vi "License Generator.vi"() -> ()   [LabVIEW 2019]
panel:
  in  "SP Generate":bool
  out "SP":string caption="Swelling Pressure"
  in  "Client MAC Address":string caption="Triaxial Shear 2"
  in  "Iso Generate":bool
  in  "UCT Generate":bool
  in  "Sat Generate":bool
  in  "Cons Generate":bool
  in  "Permeability Generate":bool
  in  "Shearbox Generate":bool
  in  "TUU Generate":bool
  in  "TS Generate":bool
  out "Isotropic":string caption="Isotropic Consolidation"
  out "UCT":string
  out "Saturation":string caption="Saturation (Incremental)"
  out "Consolidation":string caption="Consolidation (Stepped Loadning)"
  out "Permeability":string
  out "Shearbox":string
  out "Triaxial UU":string
  out "Triaxial Shear":string
  # "\"getmac\" on client command prompt"
  # "Test Type Module"
  # "Activation Code"
  # "Generate"
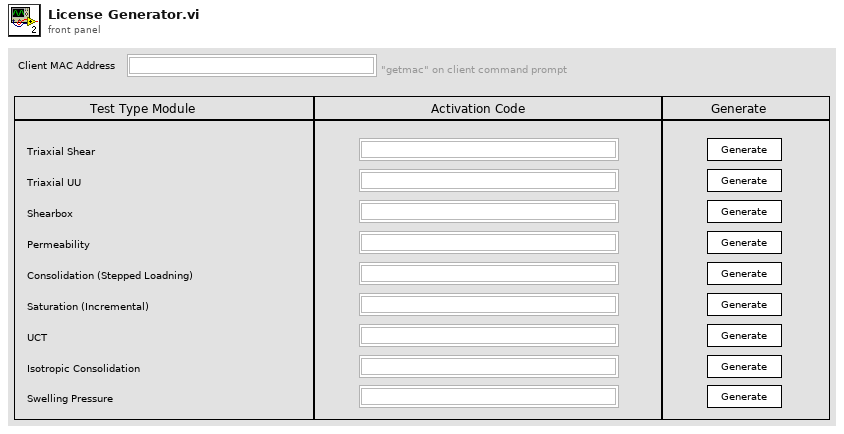
[diagram p1: front panel]
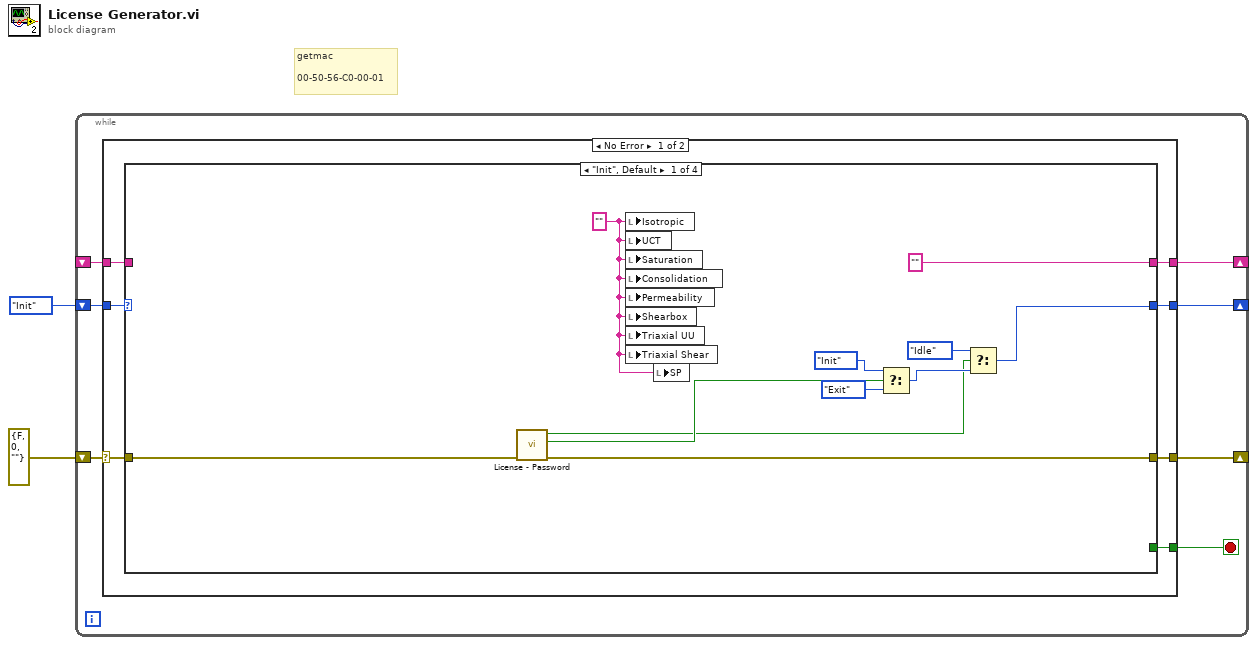
[diagram p0: block diagram]
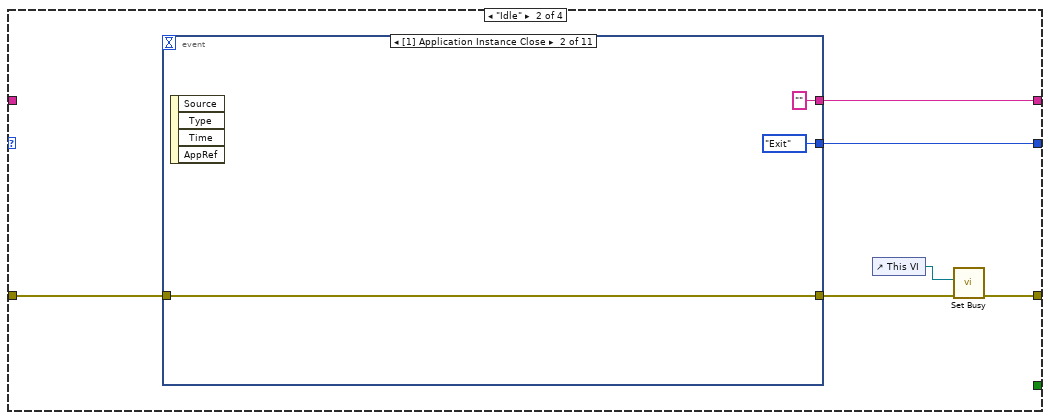
[diagram p2: hidden frame]
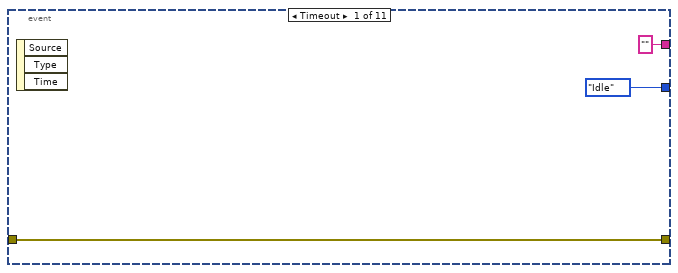
[diagram p3: hidden frame]
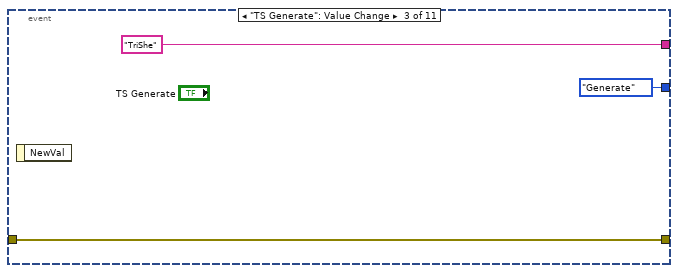
[diagram p4: hidden frame]
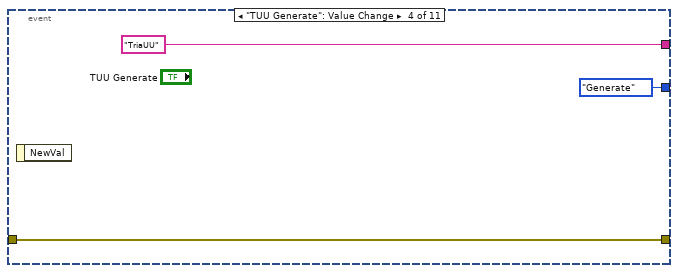
[diagram p5: hidden frame]
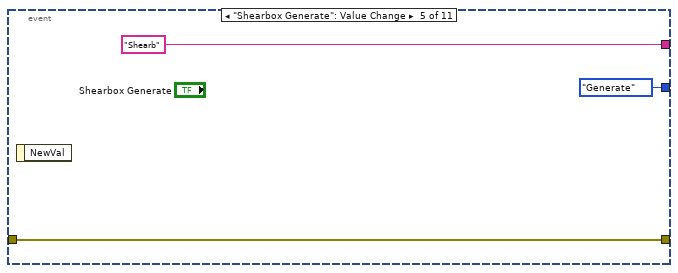
[diagram p6: hidden frame]
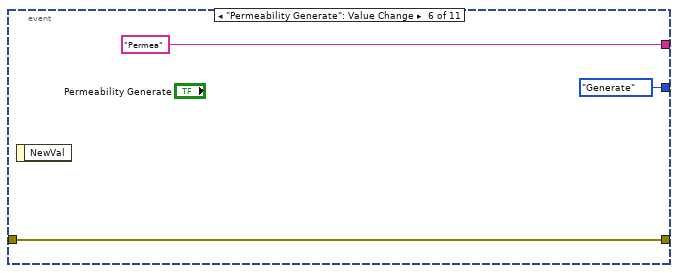
[diagram p7: hidden frame]
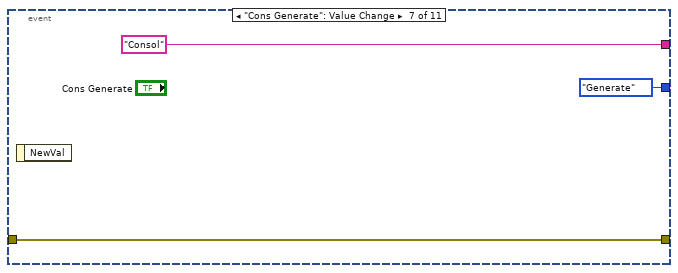
[diagram p8: hidden frame]
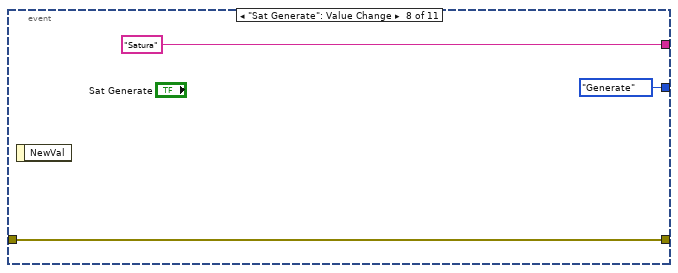
[diagram p9: hidden frame]
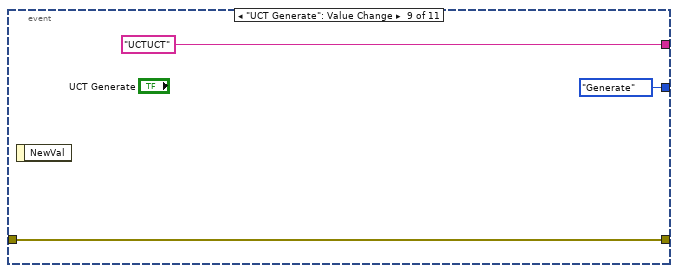
[diagram p10: hidden frame]
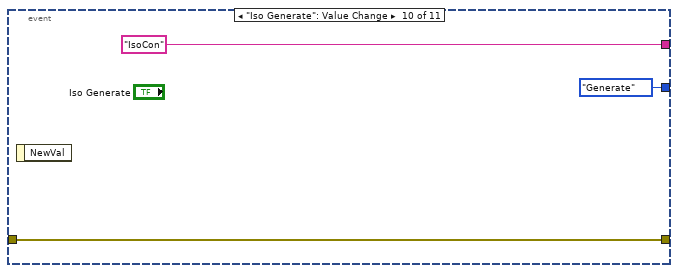
[diagram p11: hidden frame]
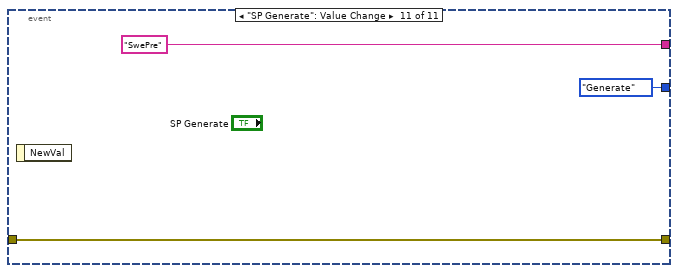
[diagram p12: hidden frame]
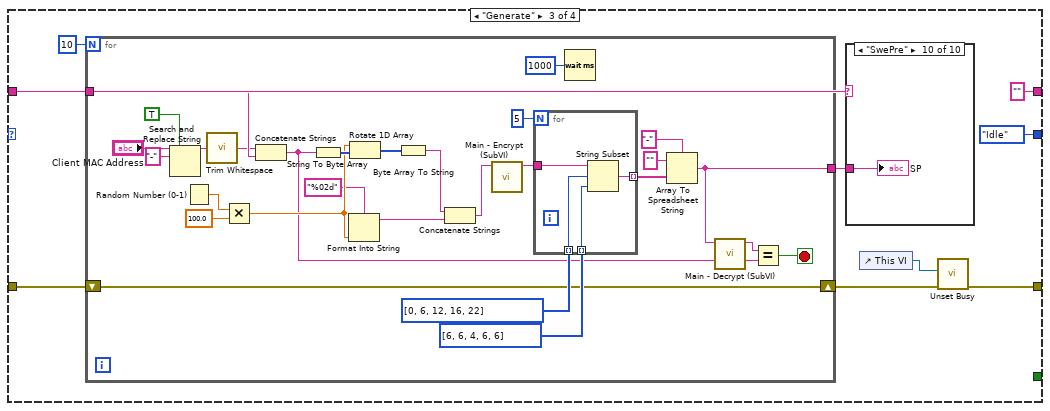
[diagram p13: hidden frame]
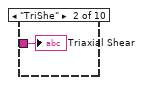
[diagram p15: hidden frame]
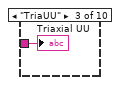
[diagram p16: hidden frame]
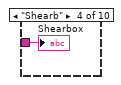
[diagram p17: hidden frame]
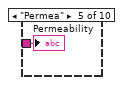
[diagram p18: hidden frame]
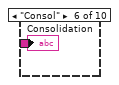
[diagram p19: hidden frame]
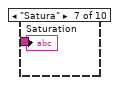
[diagram p20: hidden frame]
diagram:
  # "getmac\n\n00-50-56-C0-00-01"
  n1 = while {
    shift-right: [w6] -> _
    shift-left: enum16{"Init", "Idle", "Generate", "Exit"}."Init" -> [w9]
    shift-right: [w7] -> _
    shift-left: errorcluster {"status"=FALSE, "code"=0, "source"=""} ("error constant") -> [w8]
    shift-right: [w5] -> _
    shift-left: _ -> [w4]
    stop <- w3 stop-if-true
    n2 = case shown="No Error" w8 {
      selector: w8 -> [w14 w125]
      tunnel: w9 -> [w16 _]
      tunnel: [w15 w124] -> w7
      tunnel: [w13 enum16{"Init", "Idle", "Generate", "Exit"}."Idle"] -> w6
      tunnel: [w12 ""] -> w5
      tunnel: w4 -> [w11 _]
      tunnel: [w10 _] -> w3
      frame No Error {
        n3 = case shown="\"Init\", Default" w16 {
          tunnel: [w25 w30 w68 w120] -> w15
          tunnel: w14 -> [w24 w33 w70 w120]
          tunnel: [w17 w32 enum16{"Init", "Idle", "Generate", "Exit"}."Idle" enum16{"Init", "Idle", "Generate", "Exit"}."Exit"] -> w13
          tunnel: ["" w31 "" ""] -> w12
          tunnel: w11 -> [_ _ w73 _]
          tunnel: [_ _ _ TRUE] -> w10
          frame "Init", Default {
            w26 = "" ("Isotropic")
            n4 = call "License - Password.vi"("error in"=w24) -> ("error out"=w25:errorcluster, "T button?"=w23:bool, "Pass?"=w19:bool)  [unwired: 8 in]
            n5 = local write "Isotropic"(w26) -> ()
            n6 = local write "UCT"(w26) -> ()
            n7 = local write "Saturation"(w26) -> ()
            n8 = local write "Consolidation"(w26) -> ()
            n9 = local write "Permeability"(w26) -> ()
            n10 = local write "Shearbox"(w26) -> ()
            n11 = local write "Triaxial UU"(w26) -> ()
            n12 = local write "Triaxial Shear"(w26) -> ()
            n13 = local write "SP"(w26) -> ()
            n14 = Select(t=enum16{"Init", "Idle", "Generate", "Exit"}."Init", s=w23, f=enum16{"Init", "Idle", "Generate", "Exit"}."Exit") -> (s? t:f=w20:enum16{"Init", "Idle", "Generate", "Exit"})
            n15 = Select(t=enum16{"Init", "Idle", "Generate", "Exit"}."Idle", s=w19, f=w20) -> (s? t:f=w17:enum16{"Init", "Idle", "Generate", "Exit"})
          }
          frame "Idle" {
            n16 = event shown="[1] Application Instance Close" {
              selector: _ -> [_ _ _ _ _ _ _ _ _ _ _]
              dyn-events: _ -> [_ _ _ _ _ _ _ _ _ _ _]
              timeout: _ -> [_ _ _ _ _ _ _ _ _ _ _]
              tunnel: [w36 w39 w42 w45 w48 w51 w54 w57 w60 w63 w66] -> w29
              tunnel: w33 -> [w36 w39 w42 w45 w48 w51 w54 w57 w60 w63 w66]
              tunnel: [enum16{"Init", "Idle", "Generate", "Exit"}."Idle" enum16{"Init", "Idle", "Generate", "Exit"}."Exit" enum16{"Init", "Idle", "Generate", "Exit"}."Generate" enum16{"Init", "Idle", "Generate", "Exit"}."Generate" enum16{"Init", "Idle", "Generate", "Exit"}."Generate" enum16{"Init", "Idle", "Generate", "Exit"}."Generate" enum16{"Init", "Idle", "Generate", "Exit"}."Generate" enum16{"Init", "Idle", "Generate", "Exit"}."Generate" enum16{"Init", "Idle", "Generate", "Exit"}."Generate" enum16{"Init", "Idle", "Generate", "Exit"}."Generate" enum16{"Init", "Idle", "Generate", "Exit"}."Generate"] -> w32
              tunnel: ["" "" "TriShe" "TriaUU" "Shearb" "Permea" "Consol" "Satura" "UCTUCT" "IsoCon" "SwePre"] -> w31
              event Timeout {
                n17 = event-data() -> ()  [unwired: 1 in, 3 out]
              }
              event Application Instance Close {
                n18 = event-data() -> ()  [unwired: 1 in, 4 out]
              }
              event "TS Generate": Value Change {
                n19 = event-data() -> ()  [unwired: 1 in, 1 out]
              }
              event "TUU Generate": Value Change {
                n20 = event-data() -> ()  [unwired: 1 in, 1 out]
              }
              event "Shearbox Generate": Value Change {
                n21 = event-data() -> ()  [unwired: 1 in, 1 out]
              }
              event "Permeability Generate": Value Change {
                n22 = event-data() -> ()  [unwired: 1 in, 1 out]
              }
              event "Cons Generate": Value Change {
                n23 = event-data() -> ()  [unwired: 1 in, 1 out]
              }
              event "Sat Generate": Value Change {
                n24 = event-data() -> ()  [unwired: 1 in, 1 out]
              }
              event "UCT Generate": Value Change {
                n25 = event-data() -> ()  [unwired: 1 in, 1 out]
              }
              event "Iso Generate": Value Change {
                n26 = event-data() -> ()  [unwired: 1 in, 1 out]
              }
              event "SP Generate": Value Change {
                n27 = event-data() -> ()  [unwired: 1 in, 1 out]
              }
            }
            n28 = control-ref of="This VI"() -> (w28:refnum<vi>)
            n29 = call <vilib>:"Set Busy.vi"("error in (no error)"=w29, "VI reference (current VI)"=w28) -> ("error out"=w30:errorcluster)  [unwired: 8 in, 1 out]
          }
          frame "Generate" {
            n30 = for {
              N: 10 -> [_]
              tunnel: w73 -> [w87]
              tunnel: [w83] -> w72
              shift-right: [w77] -> w69
              shift-left: w70 -> [w77]
              stop <- w76 stop-if-true
              n31 = Search and Replace String(replace all?=TRUE ("replace all? (F)"), input string="Client MAC Address", search string="-") -> (result string=w88:string)  [unwired: 5 in, 3 out]
              n32 = Random Number (0-1)() -> (number: 0 to 1=w98:dbl)
              n33 = call <vilib>:"Trim Whitespace.vi"("string"=w88) -> ("trimmed string"=w86:string)  [unwired: 1 in]
              n34 = Multiply(x=w98, y=100.0) -> (x*y=w94:dbl)
              n35 = Concatenate Strings(w86, w87) -> (w80:string)
              n36 = String To Byte Array(string=w80) -> (unsigned byte array=w96:u8[])
              n37 = Format Into String(format string="%02d", w94) -> (resulting string=w92:string)  [unwired: 2 in, 1 out]
              n38 = Rotate 1D Array(1:w96, 2:w94) -> (0:w95:u8[])
              n39 = Byte Array To String(unsigned byte array=w95) -> (string=w79:string)
              n40 = Concatenate Strings(w79, w92) -> (w81:string)
              n41 = call "Main - Encrypt (SubVI).vi"("String"=w81) -> ("Base64 String"=w103:string)  [unwired: 10 in]
              n42 = for {
                N: 5 -> [_]
                tunnel: w103 -> [w107]
                tunnel: [w106] -> w101 mode=indexing
                tunnel: i32[] [0, 6, 12, 16, 22] ("length (rest)") -> [w105] mode=indexing
                tunnel: i32[] [6, 6, 4, 6, 6] ("length (rest)") -> [w104] mode=indexing
                n43 = String Subset(string=w107, offset (0)=w105, length (rest)=w104) -> (substring=w106:string)
              }
              n44 = Wait (ms)(milliseconds to wait=u32 1000) -> ()  [unwired: 1 out]
              n45 = Array To Spreadsheet String(delimiter (Tab)="-", array=w101, 3:"" ("format string")) -> (spreadsheet string=w83:string)
              n46 = call "Main - Decrypt (SubVI).vi"("Base64 String"=w83) -> ("String"=w82:string)  [unwired: 9 in]
              n47 = Equal?(x=w82, y=w80) -> (x = y?=w76:bool)
            }
            n48 = case shown="\"SwePre\"" w73 {
              tunnel: w72 -> [_ w108 w109 w110 w111 w112 w113 w114 w115 w116]
              frame Default {
              }
              frame "TriShe" {
                "Triaxial Shear" <- w108
              }
              frame "TriaUU" {
                "Triaxial UU" <- w109
              }
              frame "Shearb" {
                "Shearbox" <- w110
              }
              frame "Permea" {
                "Permeability" <- w111
              }
              frame "Consol" {
                "Consolidation" <- w112
              }
              frame "Satura" {
                "Saturation" <- w113
              }
              frame "UCTUCT" {
                "UCT" <- w114
              }
              frame "IsoCon" {
                "Isotropic" <- w115
              }
              frame "SwePre" {
                "SP" <- w116
              }
            }
            n49 = control-ref of="This VI"() -> (w67:refnum<vi>)
            n50 = call <vilib>:"Unset Busy.vi"("error in (no error)"=w69, "VI reference (current VI)"=w67) -> ("error out"=w68:errorcluster)  [unwired: 9 in]
          }
          frame "Exit" {
          }
        }
      }
      frame Error {
        n51 = call <vilib>:"Clear Errors.vi"("error in (no error)"=w125) -> ("error out"=w124:errorcluster)  [unwired: 5 in, 1 out]
        n52 = Wait (ms)(milliseconds to wait=u32 100) -> ()  [unwired: 1 out]
      }
    }
  }
